vi "Zoom immagine grafici.vi"(9 "image data in":T1, 10 "Zoom Factor":sgl, 11 "Picture in":refnum<vi>) -> (2 "image data out":T1)   [LabVIEW 2019]
uses:
  <vilib>/picture/picture.llb/imagedata.ctl
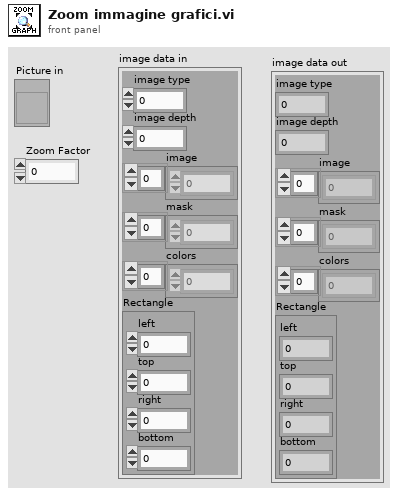
[diagram p1: front panel]
types:
  T1 = typedef "imagedata.ctl" = cluster{"image type":i32, "image depth":i32, "image":u8[], "mask":u8[], "colors":u32[], "Rectangle":cluster{"left":i16, "top":i16, "right":i16, "bottom":i16}}
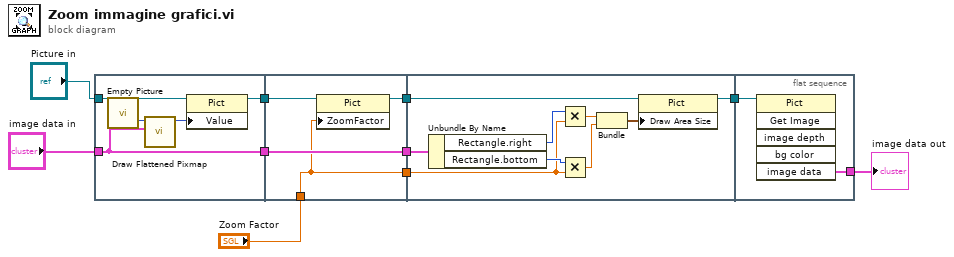
[diagram p0: block diagram]
diagram:
  n1 = flat-sequence {
    tunnel: "image data in" -> [w14]
    tunnel: [w14] -> w10
    tunnel: "Picture in" -> [w13]
    tunnel: [w12] -> w4
    tunnel: [w19] -> w9
    tunnel: w10 -> [w19]
    tunnel: [w16] -> w8
    tunnel: w4 -> [w18]
    tunnel: [w17] -> w3
    tunnel: "Zoom Factor" -> [w16]
    tunnel: w9 -> [w24]
    tunnel: w8 -> [w22]
    tunnel: w3 -> [w21]
    tunnel: [w20] -> w2
    tunnel: [w30] -> w7
    tunnel: w2 -> [w29]
    frame #0 {
      n2 = call "Empty Picture"() -> ("empty picture"=w15:picture)
      n3 = call <vilib>:"Draw Flattened Pixmap.vi"("image data"=w14, "picture"=w15) -> ("new picture"=w11:picture)  [unwired: 7 in]
      n4 = property on="Property Node" class="Pict"(reference=w13, "Value"=w11) -> (reference out=w12:refnum<vi>)  [unwired: 1 in, 1 out]
    }
    frame #1 {
      n5 = property on="Property Node" class="Pict"(reference=w18, "ZoomFactor"=w16) -> (reference out=w17:refnum<vi>)  [unwired: 1 in, 1 out]
    }
    frame #2 {
      n6 = Unbundle By Name(w24) -> ("Rectangle.right"=w27:i16, "Rectangle.bottom"=w28:i16)
      n7 = Multiply(x=w27, y=w22) -> (x*y=w25:sgl)
      n8 = Multiply(x=w28, y=w22) -> (x*y=w26:sgl)
      n9 = Bundle(w25, w26) -> (w23:cluster{sgl, sgl})  [unwired: 1 in]
      n10 = property on="Property Node" class="Pict"(reference=w21, "Draw Area Size"=w23) -> (reference out=w20:refnum<vi>)  [unwired: 1 in, 1 out]
    }
    frame #3 {
      n11 = invoke on="Invoke Node" class="Pict" method="Get Image"(reference=w29) -> ("image data"=w30:T1)  [unwired: 5 in, 5 out]
    }
  }
  "image data out" <- w7
